vi "Gradients Wavenet-IIR.vi"(1 "Wavenet-IIR Memories":T1 {"Activation functions, dF" format="%.3f"; "Wavenet, Z" format="%.3f"; "Tracking errors, e" format="%.3f"; "Activation functions, F" format="%.3f"; "Wavenet-IIR, Y" format="%.3f"}, 2 "Wavenet-IIR Values":T3 {"Function, dy" format="%.3f"; "Function, y" format="%.3f"; "Tau, t" format="%.3f"; "Forwards, D" format="%.3f"; "Feedbacks, C" format="%.3f"; "Weights, W" format="%.3f"; "Shifts, B" format="%.3f"; "Scales, A" format="%.3f"}, 3 "Pitch, e":dbl=1.0 format="%.2f", 4 "Yaw, e":dbl=1.0 format="%.2f", 5 "Persistant signal":dbl format="%.2e", 6 "Total control, U":dbl=1.0 format="%.3f") -> (0 "Wavenet-IIR Gradients":T2 {"Forwards, D" format="%.3f"; "Feedbacks, C" format="%.3f"; "Weights, W" format="%.3f"; "Shifts, B" format="%.3f"; "Scales, A" format="%.3f"})   [LabVIEW 2022 SP3]
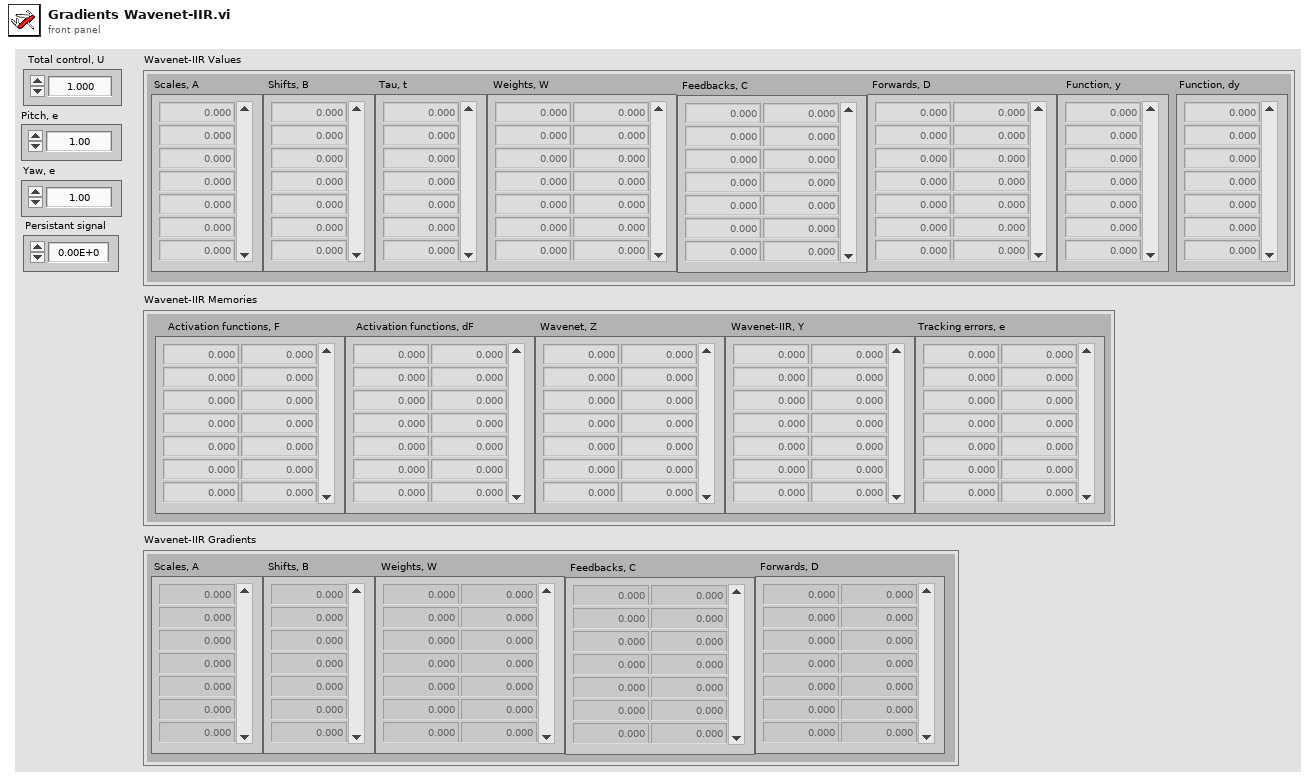
[diagram p1: front panel]
types:
  T1 = cluster{"Wavenet-IIR, Y":dbl[][], "Activation functions, F":dbl[][], "Tracking errors, e":dbl[][], "Wavenet, Z":dbl[][], "Activation functions, dF":dbl[][]}
  T2 = cluster{"Scales, A":dbl[], "Shifts, B":dbl[], "Weights, W":dbl[][], "Feedbacks, C":dbl[][], "Forwards, D":dbl[][]}
  T3 = cluster{"Scales, A":dbl[], "Shifts, B":dbl[], "Weights, W":dbl[][], "Feedbacks, C":dbl[][], "Forwards, D":dbl[][], "Tau, t":dbl[], "Function, y":dbl[], "Function, dy":dbl[]}
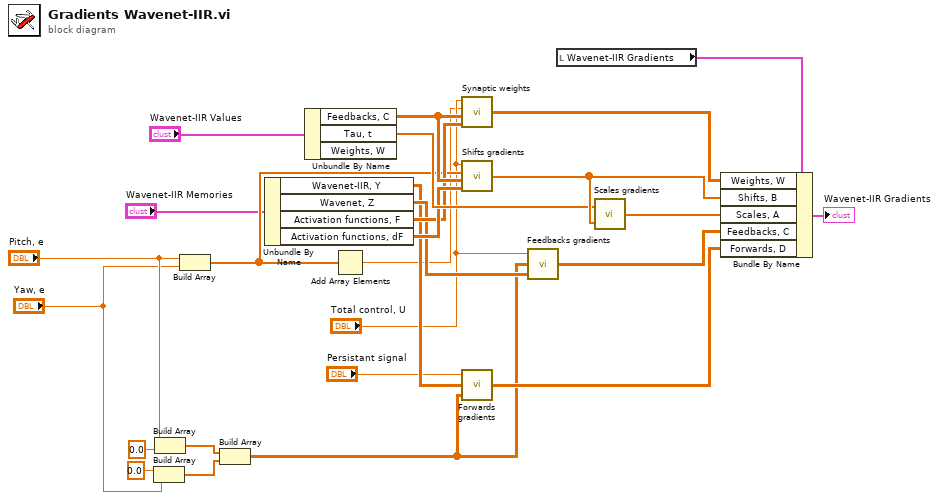
[diagram p0: block diagram]
diagram:
  n1 = Build Array(0.0 ("element"), "Yaw, e") -> (w2:dbl[])
  n2 = Build Array("Pitch, e", 0.0 ("element")) -> (w3:dbl[])
  n3 = Build Array("Pitch, e", "Yaw, e") -> (w11:dbl[])
  n4 = Build Array(w3, w2) -> (w1:dbl[][])
  n5 = Unbundle By Name("Wavenet-IIR Memories") -> ("Wavenet-IIR, Y"=w14:dbl[][], "Wavenet, Z"=w16:dbl[][], "Activation functions, F"=w20:dbl[][], "Activation functions, dF"=w23:dbl[][])
  n6 = Unbundle By Name("Wavenet-IIR Values") -> ("Feedbacks, C"=w22:dbl[][], "Tau, t"=w24:dbl[])  [unwired: 1 out]
  n7 = Add Array Elements(numeric array=w11) -> (sum=w9:dbl)
  n8 = call "Synaptic weights.vi"("Activation functions, F"=w20, "Feedbacks, C"=w22, "Total error, e"=w9, "Total control, u"="Total control, U") -> ("Weights, W"=w21:dbl[][])
  n9 = call "Shifts gradients.vi"("Activation functions, dF"=w23, "Feedbacks, C"=w22, "Errors"=w11, "Total control, U"="Total control, U") -> ("Shifts, B"=w25:dbl[])
  n10 = call "Forwards gradients.vi"("Identification errors, e"=w1, "Wavenet-IIR, Y"=w14, "Persistent signal"="Persistant signal") -> ("Forwards, D"=w13:dbl[][])
  n11 = call "Feedbacks gradients.vi"("Wavenet, Z"=w16, "Identification errors, e"=w1, "Total control, U"="Total control, U") -> ("Feedbacks, C"=w15:dbl[][])
  n12 = local read "Wavenet-IIR Gradients"() -> (w18:T2)
  n13 = call "Scales gradients.vi"("Shifts, B"=w25, "Tau, t"=w24) -> ("Scales, A"=w26:dbl[])
  n14 = Bundle By Name(cluster=w18, "Weights, W"=w21, "Shifts, B"=w25, "Scales, A"=w26, "Feedbacks, C"=w15, "Forwards, D"=w13) -> (→"Wavenet-IIR Gradients":T2)
